vi "Table_根据窗格自动缩放.vi"(8 "error in (no error)":errorcluster caption="错误输入（无错误）") -> (0 "error out":errorcluster caption="错误输出")   [LabVIEW 2018]
uses:
  <vilib>/Utility/miscctls.llb/LVRowAndColumnTypeDef.ctl
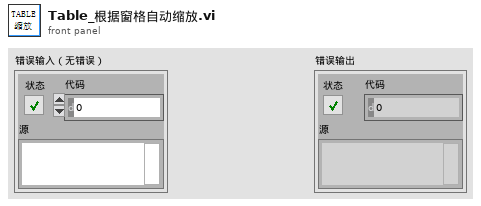
[diagram p1: front panel]
types:
  T1 = typedef "LVRowAndColumnTypeDef.ctl" = cluster{"Row":i32, "Column":i32}
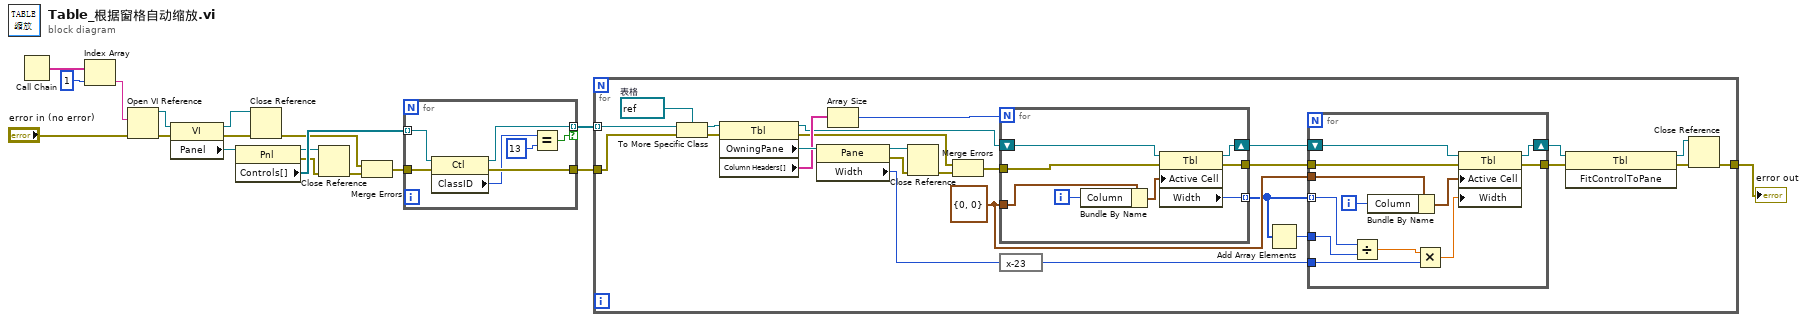
[diagram p0: block diagram]
diagram:
  n1 = Call Chain() -> (call chain=w18:string[])
  n2 = Index Array(array=w18, index=1 ("索引")) -> (element=w16:string)
  n3 = Open VI Reference(vi path=w16, error in (no error)="error in (no error)") -> (vi reference=w15:refnum<vi>, error out=w14:errorcluster)  [unwired: 4 in]
  n4 = property class="VI"(reference=w15, error in=w14) -> (reference out=w6:refnum<vi>, error out=w5:errorcluster, "Panel"=w12:refnum<vi>)
  n5 = property class="Pnl"(reference=w12) -> (reference out=w7:refnum<vi>, error out=w8:errorcluster, "Controls[]"=w11:refnum<vi>[])  [unwired: 1 in]
  n6 = Close Reference(reference=w6, error in (no error)=w5) -> (error out=w4:errorcluster)
  n7 = Close Reference(reference=w7, error in (no error)=w8) -> (error out=w3:errorcluster)
  n8 = Merge Errors(w4, w3) -> (w2:errorcluster)
  n9 = for {
    tunnel: w11 -> [w25] mode=indexing
    tunnel: [w23] -> w10 mode=indexing if=w22
    tunnel: w2 -> [w21]
    tunnel: [w20] -> w1
    n10 = property class="Ctl"(reference=w25, error in=w21) -> (reference out=w23:refnum<vi>, error out=w20:errorcluster, "ClassID"=w19:u32)
    n11 = Equal?(x=w19, y=u32 13) -> (x = y?=w22:bool)
  }
  n12 = for {
    tunnel: w10 -> [w51] mode=indexing
    tunnel: [w32] -> w9
    tunnel: w1 -> [w26]
    w39 = T1 {"Row"=0, "Column"=0} ("活动单元格:活动单元格")
    w48 = refnum<vi> refnum  # 表格
    n13 = To More Specific Class(target class=w48, reference=w51, error in=w26) -> (specific class reference=w50:refnum<vi>, error out=w49:errorcluster)
    n14 = property class="Tbl"(reference=w50, error in=w49) -> (reference out=w45:refnum<vi>, error out=w29:errorcluster, "OwningPane"=w47:refnum<vi>, "Column Headers[]"=w46:string[])
    n15 = property class="Pane"(reference=w47) -> (reference out=w31:refnum<vi>, error out=w30:errorcluster, "Width"=w36:u32)  [unwired: 1 in]
    n16 = Array Size(array=w46) -> (size(s)=w44:i32)
    n17 = Close Reference(reference=w31, error in (no error)=w30) -> (error out=w28:errorcluster)
    n18 = Merge Errors(w29, w28) -> (w27:errorcluster)
    n19 = for {
      N: w44 -> [_]
      tunnel: w39 -> [w70]
      tunnel: w27 -> [w67]
      tunnel: [w66] -> w38 mode=indexing
      tunnel: [w65] -> w43
      shift-right: [w64] -> w42
      shift-left: w45 -> [w71]
      i -> [w68]
      n20 = Bundle By Name(cluster=w70, "Column"=w68) -> (w69:T1)
      n21 = property class="Tbl"(reference=w71, error in=w67, "Active Cell"=w69) -> (reference out=w64:refnum<vi>, error out=w65:errorcluster, "Width"=w66:u32)
    }
    n22 = expression code="x-23"(w36) -> (w35:u32)
    n23 = Add Array Elements(numeric array=w38) -> (sum=w37:u32)
    n24 = for {
      tunnel: w39 -> [w62]
      tunnel: w43 -> [w59]
      shift-right: [w58] -> w41
      shift-left: w42 -> [w63]
      tunnel: [w57] -> w40
      tunnel: w38 -> [w56] mode=indexing
      tunnel: w37 -> [w55]
      tunnel: w35 -> [w53]
      i -> [w60]
      n25 = Divide(x=w56, y=w55) -> (x/y=w54:dbl)
      n26 = Bundle By Name(cluster=w62, "Column"=w60) -> (w61:T1)
      n27 = Multiply(x=w54, y=w53) -> (x*y=w52:dbl)
      n28 = property class="Tbl"(reference=w63, error in=w59, "Active Cell"=w61, "Width"=w52) -> (reference out=w58:refnum<vi>, error out=w57:errorcluster)
    }
    n29 = invoke class="Tbl" method="FitControlToPane"(reference=w41, error in=w40) -> (reference out=w34:refnum<vi>, error out=w33:errorcluster)  [unwired: 1 in, 1 out]
    n30 = Close Reference(reference=w34, error in (no error)=w33) -> (error out=w32:errorcluster)
  }
  "error out" <- w9
